vi "PWM_Lenkung_Überholen.vi"(0 "vorne rechts":dbl, 1 "vorne links":dbl, 2 "hinten rechts":dbl, 3 "hinten links":dbl, 5 "Position Strecke":dbl) -> (11 "Abstand Bande erreicht":bool, 14 "PWM Lenkung":dbl)   [LabVIEW 2016]
doc: "PID Regelung für Servowert\n05.04.17_Tloe"
uses:
  <vilib>/addons/control/pid/pid.llb/PID (DBL).vi
  <vilib>/addons/control/pid/NI_PID_pid.lvlib
panel:
  in  "PID":T1={"proportional gain (Kc)"=0.8, "integral time (Ti, min)"=0.0, "derivative time (Td, min)"=0.001} {"proportional gain (Kc)" format="%#_10g"; "integral time (Ti, min)" format="%#_10g"; "derivative time (Td, min)" format="%#_10g"}
  # "0.8"
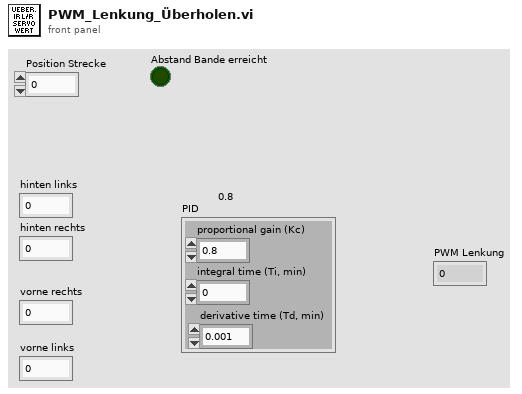
[diagram p1: front panel]
types:
  T1 = cluster{"proportional gain (Kc)":dbl, "integral time (Ti, min)":dbl, "derivative time (Td, min)":dbl}
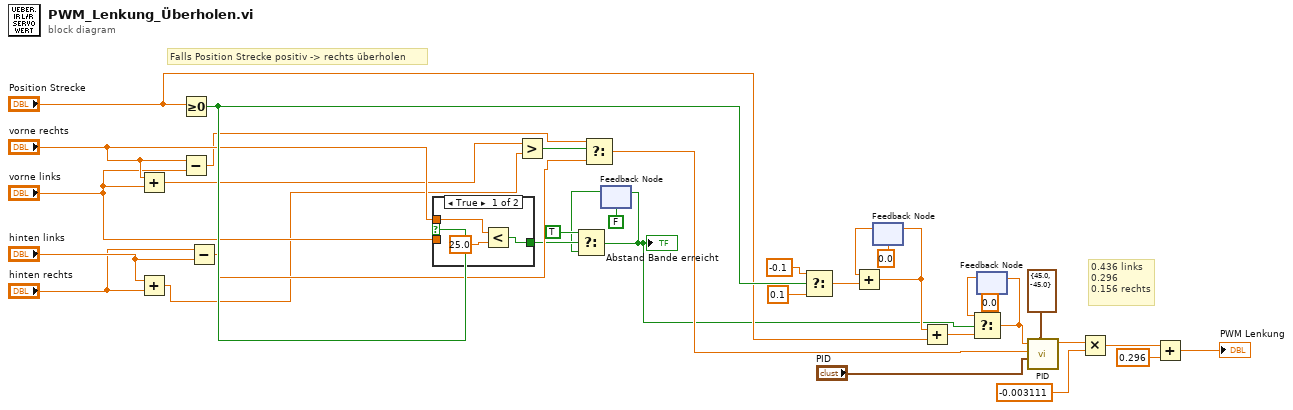
[diagram p0: block diagram]
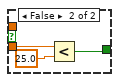
[diagram p2: hidden frame]
diagram:
  # "Falls Position Strecke positiv -> rechts überholen"
  # "0.436 links\n0.296\n0.156 rechts"
  n1 = Add(x="vorne rechts", y="vorne links") -> (x+y=w12:dbl)
  n2 = Add(x="hinten links", y="hinten rechts") -> (x+y=w11:dbl)
  n3 = Greater Or Equal To 0?(x="Position Strecke") -> (x >= 0?=w32:bool)
  n4 = Subtract(x="vorne rechts", y="vorne links") -> (x-y=w14:dbl)
  n5 = Subtract(x="hinten rechts", y="hinten links") -> (x-y=w15:dbl)
  n6 = case shown="True" w32 {
    tunnel: "vorne links" -> [_ w39]
    tunnel: "vorne rechts" -> [w36 _]
    tunnel: [w35 w38] -> w4
    frame True {
      n7 = Less?(x=w36, y=25.0) -> (x < y?=w35:bool)
    }
    frame False {
      n8 = Less?(x=w39, y=25.0) -> (x < y?=w38:bool)
    }
  }
  n9 = Greater?(x=w12, y=w11) -> (0:w31:bool)
  n10 = Select(t=w14, s=w31, f=w15) -> (s? t:f=w30:dbl)
  n11 = feedback #1(FALSE ("t")) -> (w3:bool)
  n12 = Select(t=TRUE, s=w4, f=w3) -> (s? t:f=w1:bool)
  "Abstand Bande erreicht" <- w1
  n13 = feedback-in #1(w1) -> ()
  n14 = Select(t=-0.1, s=w32, f=0.1) -> (s? t:f=w23:dbl)
  n15 = feedback #2(0.0 ("t")) -> (w29:dbl)
  n16 = Add(x=w29, y=w23) -> (x+y=w5:dbl)
  n17 = feedback-in #2(w5) -> ()
  n18 = Add(x=w5, y="Position Strecke") -> (x+y=w20:dbl)
  n19 = feedback #3(0.0) -> (w18:dbl)
  n20 = Select(t=w18, s=w1, f=w20) -> (s? t:f=w19:dbl)
  n21 = feedback-in #3(w19) -> ()
  n22 = call-poly <vilib>:"PID.vi"("output range"=cluster{"output high":dbl, "output low":dbl} {"output high"=45.0, "output low"=-45.0}, "PID gains"="PID", "process variable"=w30, "setpoint"=w19) -> ("output"=w25:dbl)  [unwired: 6 in, 1 out]
  n23 = Multiply(x=w25, y=-0.003111) -> (x*y=w26:dbl)
  n24 = Add(x=w26, y=0.296) -> (x+y=→"PWM Lenkung":dbl)
